vi "Intensity.vi"() -> ()   [LabVIEW 2020]
panel:
  in  "Stop":bool
  out "Intensity Chart":dbl[][](graph)
  in  "Custom Marker Colors":u32[](array[colorbox])=[16714752, 16860, 6618880]
  in  "IntensiveData":dbl[][](array[numeric])=[[45.0, 1.0, 90.0], [90.0, 28.0, 40.0], [45.0, 100.0, 60.0], [100.0, 20.0, 70.0]]
  out "Intensity Graph":dbl[][](graph)
  # "90"
  # "40"
  # "60"
  # "70"
  # "1"
  # "28"
  # "100"
  # "20"
  # "45"
  # "90"
  # "45"
  # "100"
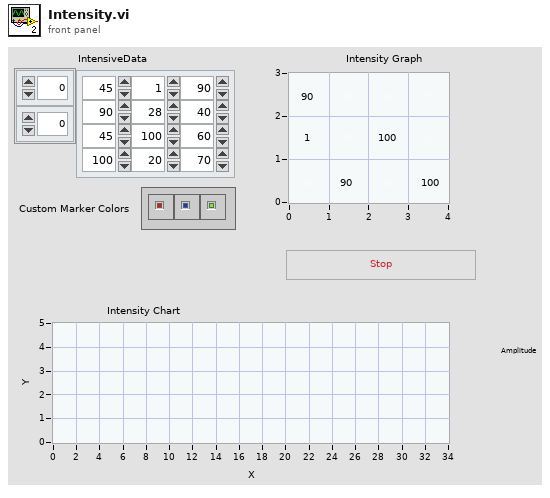
[diagram p1: front panel]
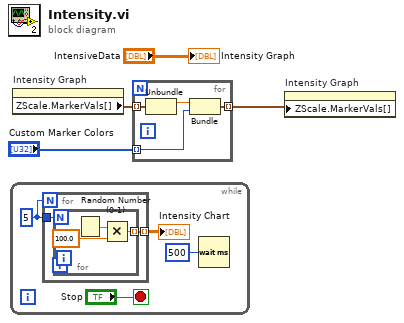
[diagram p0: block diagram]
diagram:
  n1 = while {
    stop <- "Stop" stop-if-true
    w8 = 5
    n2 = for {
      N: w8 -> [_]
      tunnel: w8 -> [w10]
      tunnel: [w9] -> w7 mode=indexing
      n3 = for {
        N: w10 -> [_]
        tunnel: [w11] -> w9 mode=indexing
        n4 = Random Number (0-1)() -> (number: 0 to 1=w13:dbl)
        n5 = Multiply(x=w13, y=100.0) -> (x*y=w11:dbl)
      }
    }
    "Intensity Chart" <- w7
    n6 = Wait (ms)(milliseconds to wait=u32 500) -> ()  [unwired: 1 out]
  }
  n7 = property on="Intensity Graph" class="IntGraph (strict)"() -> ("ZScale.MarkerVals[]"=w3:cluster{dbl, u32}[])  [unwired: 2 in, 2 out]
  n8 = for {
    tunnel: w3 -> [w17] mode=indexing
    tunnel: "Custom Marker Colors" -> [w15] mode=indexing
    tunnel: [w14] -> w2 mode=indexing
    n9 = Unbundle(w17) -> (w16:dbl)  [unwired: 1 out]
    n10 = Bundle(w16, "Color Box"=w15) -> (w14:cluster{dbl, "Color Box":u32})  [unwired: 1 in]
  }
  n11 = property on="Intensity Graph" class="IntGraph (strict)"("ZScale.MarkerVals[]"=w2) -> ()  [unwired: 2 in, 2 out]
  "Intensity Graph" <- "IntensiveData"
